vi "GetSide.vi"(8 "error in (no error)":errorcluster, 10 "Direction":T1, 11 "Room in":refnum<class "Room.lvclass">) -> (0 "error out":errorcluster, 2 "MapSite*":refnum<data-value>, 3 "Room out":refnum<class "Room.lvclass">)   [LabVIEW 2016, in "Room.lvclass"]
uses:
  Room.lvclass
  MapSite/MapSite.lvclass
  Direction.ctl
  Room.lvclass/Room.ctl
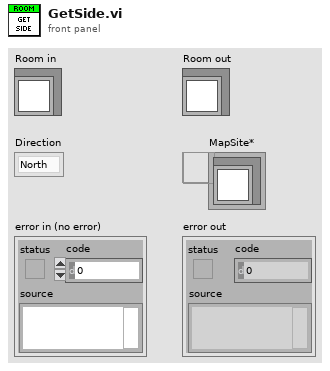
[diagram p1: front panel]
types:
  T1 = typedef "Room.lvclass/Direction.ctl" = enum16{"North", "South", "East", "West"}
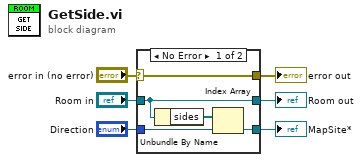
[diagram p0: block diagram]
diagram:
  n1 = case shown="No Error" "error in (no error)" {
    selector: "error in (no error)" -> [w11 w13]
    tunnel: [w11 w13] -> w5
    tunnel: [w10 w12] -> w3
    tunnel: "Room in" -> [w10 w12]
    tunnel: "Direction" -> [w8 _]
    tunnel: [w7 _] -> w1
    frame No Error {
      n2 = Unbundle By Name(w10) -> ("sides"=w9:refnum<data-value>[])
      n3 = Index Array(array=w9, index=w8) -> (element=w7:refnum<data-value>)
    }
    frame Error {
    }
  }
  "error out" <- w5
  "Room out" <- w3
  "MapSite*" <- w1
